vi "read TBM configuration.vi"(8 "error in":errorcluster, 11 "Temperature Controller Logic editor node in":refnum<class "Temperature Controller Logic editor node.lvclass">) -> (0 "error out":errorcluster, 2 "configuration":refnum<class "TBM configuration.lvclass">, 3 "Temperature Controller Logic editor node out":refnum<class "Temperature Controller Logic editor node.lvclass">)   [LabVIEW 2013, in "Temperature Controller Logic editor node.lvclass"]
uses:
  Temperature Controller Logic editor node.lvclass
  <vilib>/NI/Tag Bus Module Framework/root configuration/TBM configuration.lvclass
  Temperature Controller Logic editor node.lvclass/Temperature Controller Logic editor node.ctl
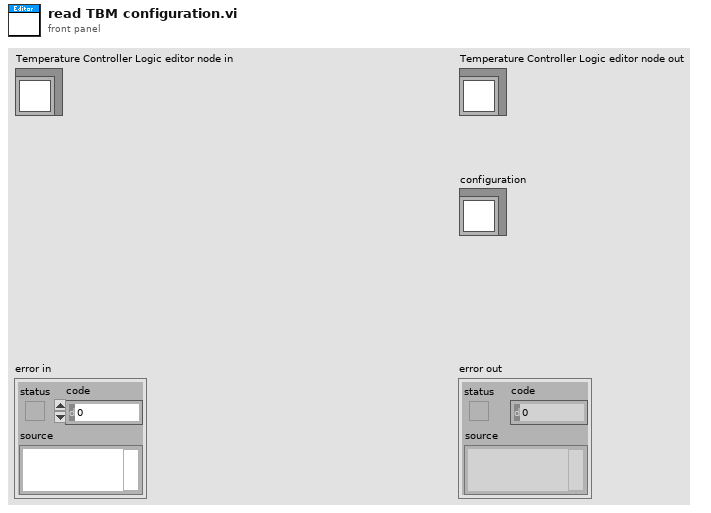
[diagram p1: front panel]
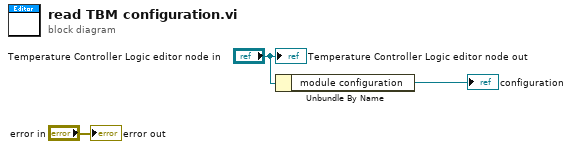
[diagram p0: block diagram]
diagram:
  n1 = Unbundle By Name("Temperature Controller Logic editor node in") -> ("module configuration"=→"configuration":refnum<class "Temperature Controller Logic configuration.lvclass">)
  "error out" <- "error in"
  "Temperature Controller Logic editor node out" <- "Temperature Controller Logic editor node in"
